vi "7.3-Create OCU to Forebrain Neuron.vi"() -> (0 "output cluster":T1={"6.1 Act"={"6.1-Saitek Controller"={"Stop"=FALSE, "Setpoint"=FALSE, "Run"=FALSE, "Restart"=FALSE, "Shutdown"=FALSE, "Joystick\nMode 1"=FALSE, "Joystick\nMode 2"=FALSE, "Joystick \nMode 3"=TRUE, "Joystick Mode 4"=FALSE, "10"=FALSE, "11"=FALSE, "Pitch"=0.0019531846, "Roll"=-0.0019531846, "Yaw"=-0.007812738, "Left"=0.828135, "Right"=0.81250954}, "Joystick Mode"=TRUE, "Shutdown"=FALSE, "Reset"=FALSE, "Begin"=FALSE}, "7.6 - GPS Waypoints Data"={"GPS Waypoint Center (Lat, Long)"=[], "5.1.1 MDF GPS"=[]}} {"6.1 Act"."6.1-Saitek Controller"."Right" scale=0.0..1.0; "6.1 Act"."6.1-Saitek Controller"."Left" scale=0.0..1.0; "6.1 Act"."6.1-Saitek Controller"."Yaw" scale=-1.0..1.0; "6.1 Act"."6.1-Saitek Controller"."Roll" scale=-1.0..1.0; "6.1 Act"."6.1-Saitek Controller"."Pitch" scale=-1.0..1.0; "7.6 - GPS Waypoints Data"."5.1.1 MDF GPS"."Latitude (waypoint)" format="%#_8g"; "7.6 - GPS Waypoints Data"."5.1.1 MDF GPS"."Longitude  (waypoint)" format="%#_8g"})   [LabVIEW 2010]
uses:
  6-OCU Neurons/6.0-OCU to Forebrain Neuron.ctl
  6-OCU Neurons/6.1-Act.ctl
  6-OCU Neurons/6.1-UDP Saitek.ctl
  7.6 - GPS Waypoint Def.ctl
  6-OCU Neurons/MDF Array LatLong.ctl
  6-OCU Neurons/MDF LatLong.ctl
  7.0-Global.vi
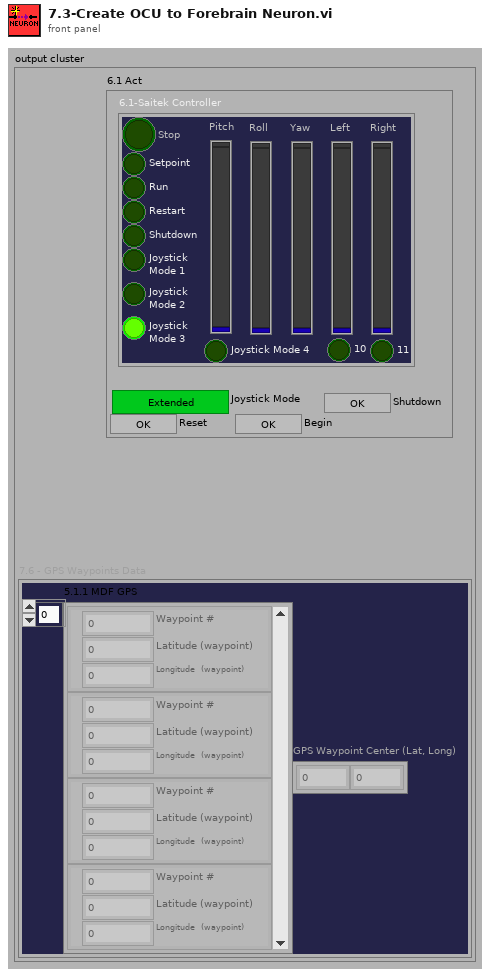
[diagram p1: front panel]
types:
  T1 = typedef "6.0-OCU to Forebrain Neuron.ctl" = cluster{"6.1 Act":T2, "7.6 - GPS Waypoints Data":T4}
  T2 = typedef "6.1-Act.ctl" = cluster{"6.1-Saitek Controller":T3, "Joystick Mode":bool, "Shutdown":bool, "Reset":bool, "Begin":bool}
  T3 = typedef "6.1-UDP Saitek.ctl" = cluster{"Stop":bool, "Setpoint":bool, "Run":bool, "Restart":bool, "Shutdown":bool, "Joystick\nMode 1":bool, "Joystick\nMode 2":bool, "Joystick \nMode 3":bool, "Joystick Mode 4":bool, "10":bool, "11":bool, "Pitch":sgl, "Roll":sgl, "Yaw":sgl, "Left":sgl, "Right":sgl}
  T4 = typedef "7.6 - GPS Waypoint Def.ctl" = cluster{"GPS Waypoint Center (Lat, Long)":dbl[], "5.1.1 MDF GPS":T5}
  T5 = typedef "MDF Array LatLong.ctl" = T6[]
  T6 = typedef "MDF LatLong.ctl" = cluster{"Waypoint #":dbl, "Latitude (waypoint)":ext, "Longitude  (waypoint)":ext}
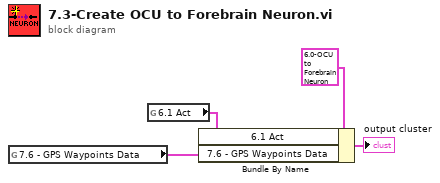
[diagram p0: block diagram]
diagram:
  n1 = global read "7.0-Global.vi" "7.6 - GPS Waypoints Data"() -> (w3:T4)
  n2 = global read "7.0-Global.vi" "6.1 Act"() -> (w4:T2)
  n3 = Bundle By Name(cluster=T1 {"6.1 Act"={"6.1-Saitek Controller"={"Stop"=FALSE, "Setpoint"=FALSE, "Run"=FALSE, "Restart"=FALSE, "Shutdown"=FALSE, "Joystick\nMode 1"=FALSE, "Joystick\nMode 2"=FALSE, "Joystick \nMode 3"=TRUE, "Joystick Mode 4"=FALSE, "10"=FALSE, "11"=FALSE, "Pitch"=0.0019531846, "Roll"=-0.0019531846, "Yaw"=-0.007812738, "Left"=0.828135, "Right"=0.81250954}, "Joystick Mode"=TRUE, "Shutdown"=FALSE, "Reset"=FALSE, "Begin"=FALSE}, "7.6 - GPS Waypoints Data"={"GPS Waypoint Center (Lat, Long)"=[], "5.1.1 MDF GPS"=[]}} ("input cluster"), "6.1 Act"=w4, "7.6 - GPS Waypoints Data"=w3) -> (→"output cluster":T1)
